vi "HoldLift.vi"(10 "Requested Lift position":dbl) -> (2 "Lift position out":dbl)   [LabVIEW 2017]
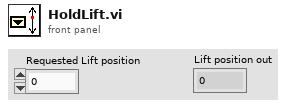
[diagram p1: front panel]
types:
  T1 = typedef "WPI_DriverStationRobotMode2.ctl" = enum16{"Autonomous Disabled", "Autonomous Enabled", "Teleop Disabled", "Teleop Enabled", "Disconnected", "Finish", "Test Disabled", "Test Enabled", "Emergency Stopped"}
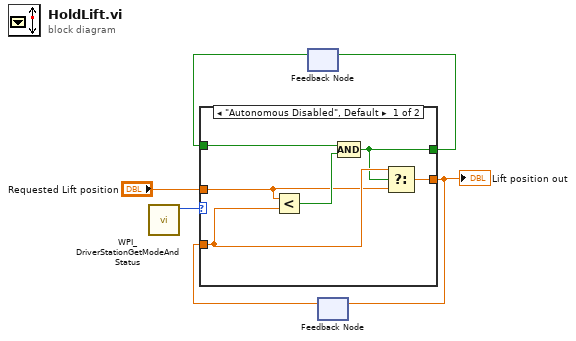
[diagram p0: block diagram]
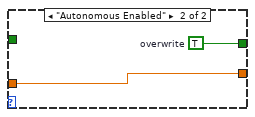
[diagram p2: hidden frame]
diagram:
  n1 = call <vilib>:"WPI_DriverStationGetModeAndStatus.vi"() -> ("Robot Mode"=w6:T1)  [unwired: 10 in, 1 out]
  n2 = feedback #1() -> (w1:bool)  [unwired: 1 in]
  n3 = feedback #2() -> (w4:dbl)  [unwired: 1 in]
  n4 = case shown="\"Autonomous Disabled\", Default" w6 {
    tunnel: [w11 w14] -> w3
    tunnel: "Requested Lift position" -> [w7 w14]
    tunnel: w4 -> [w9 _]
    tunnel: w1 -> [w12 _]
    tunnel: [w8 w13] -> w2
    frame "Autonomous Disabled", Default {
      n5 = Less?(x=w7, y=w9) -> (x < y?=w10:bool)
      n6 = Compound Arithmetic op=AND(w12, w10) -> (w8:bool)
      n7 = Select(t=w9, s=w8, f=w7) -> (s? t:f=w11:dbl)
    }
    frame "Autonomous Enabled" {
      w13 = TRUE  # overwrite
    }
  }
  "Lift position out" <- w3
  n8 = feedback-in #1(w2) -> ()
  n9 = feedback-in #2(w3) -> ()
